vi "Lv_DEMO.vi"() -> ()   [LabVIEW 2019]
uses:
  C:/Users/Way/source/repos/MACOs.JY.ActorFramework/examples/Lv_DEMO/TestService.dll
  TestService.dll
  C:/Users/Way/source/repos/MACOs.JY.ActorFramework/examples/Lv_DEMO/MACOs.JY.ActorFramework.Implement.NetMQ.dll
  MACOs.JY.ActorFramework.Implement.NetMQ.dll
  C:/Users/Way/source/repos/MACOs.JY.ActorFramework/examples/net472_DEMO/bin/Debug/MACOs.JY.ActorFramework.Core.dll
  net472_DEMO/bin/Debug/MACOs.JY.ActorFramework.Core.dll
  C:/Users/Way/source/repos/MACOs.JY.ActorFramework/examples/net472_DEMO/bin/Debug/MACOs.JY.ActorFramework.Clients.dll
  net472_DEMO/bin/Debug/MACOs.JY.ActorFramework.Clients.dll
panel:
  out "error out":errorcluster
  in  "stop":bool
  in  "OK Button":bool
  out "Output String":string
  in  "Input String":string
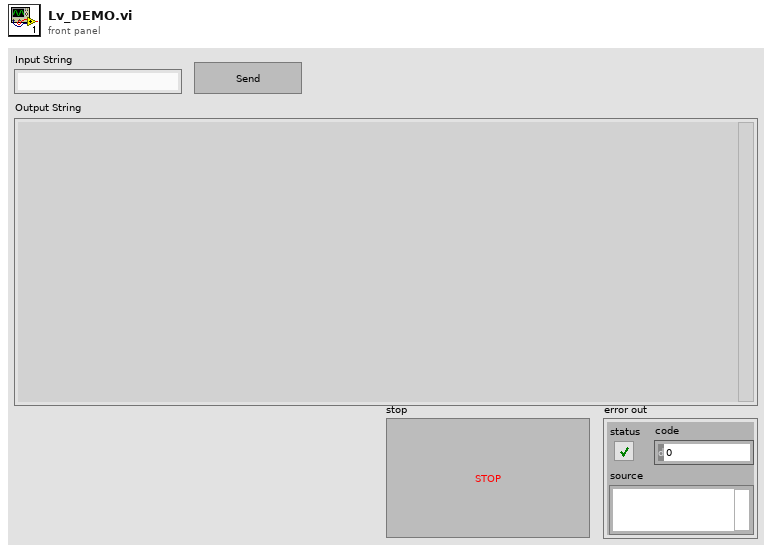
[diagram p1: front panel]
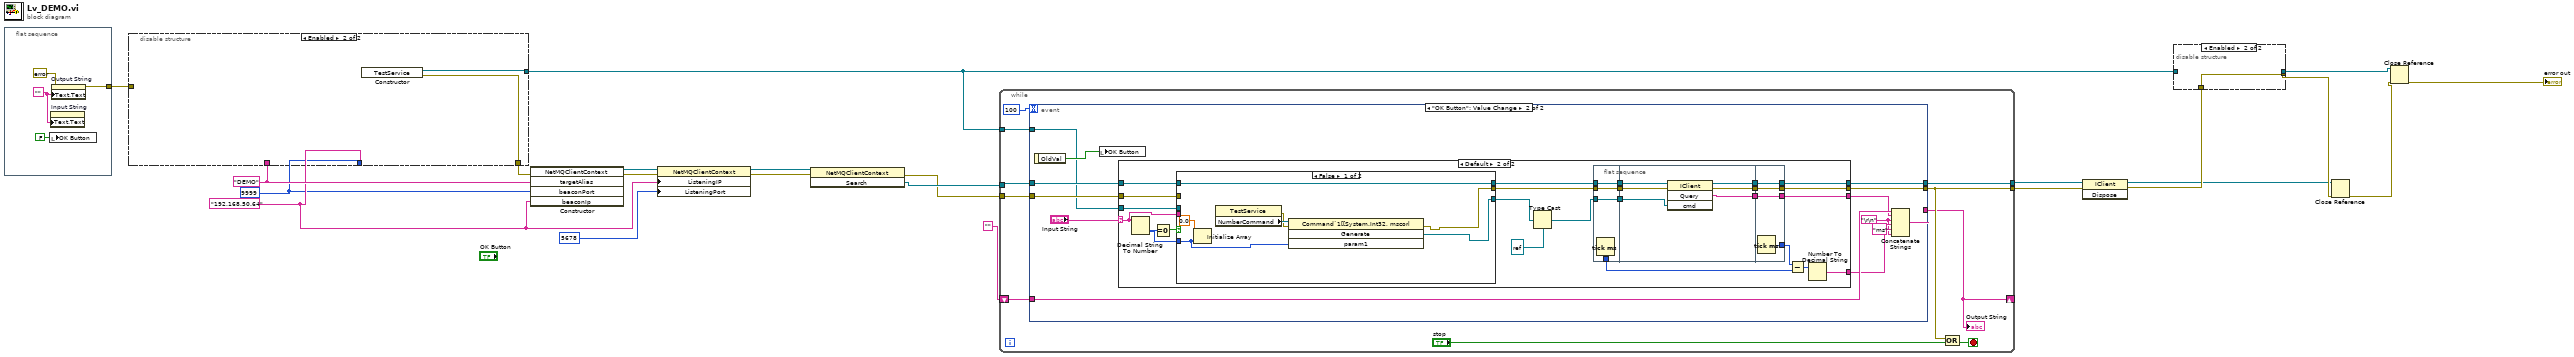
[diagram p0: block diagram]
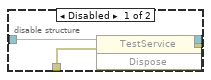
[diagram p2: hidden frame]
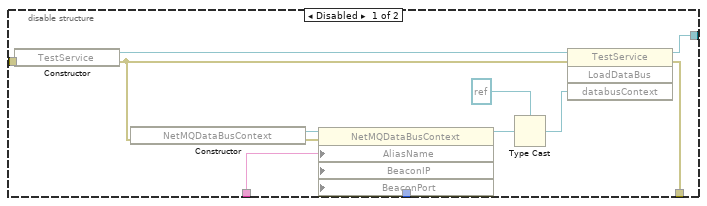
[diagram p3: hidden frame]
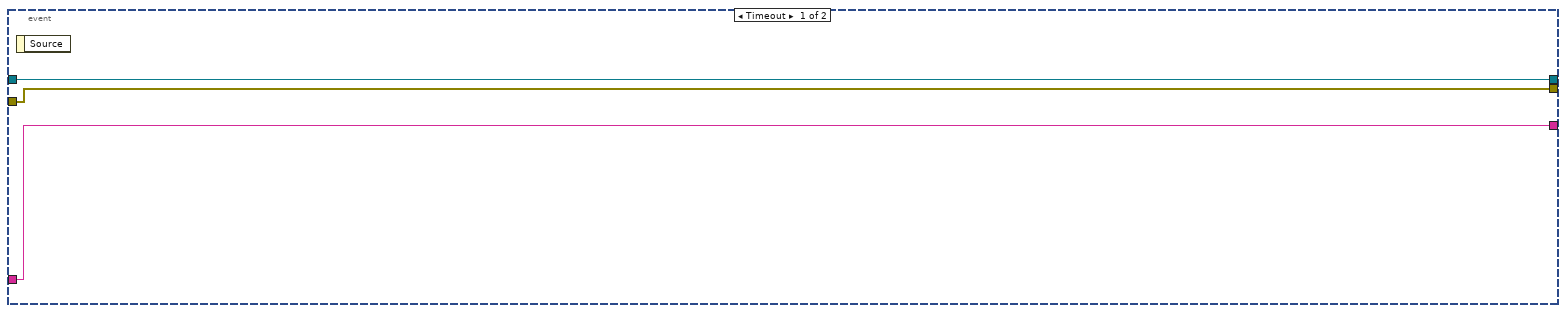
[diagram p4: hidden frame]
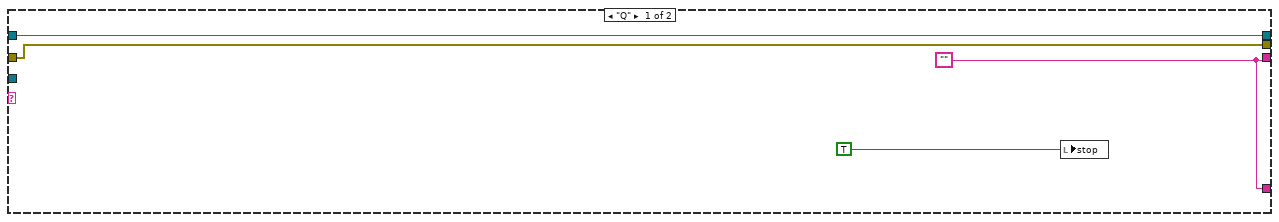
[diagram p5: hidden frame]
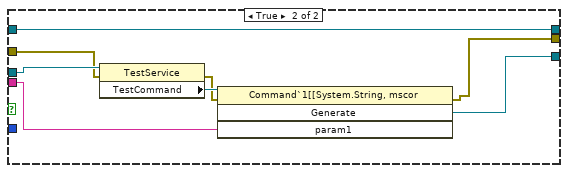
[diagram p6: hidden frame]
diagram:
  w2 = "192.168.50.64" ("alias")
  w11 = "DEMO" ("alias")
  w1 = 9999 ("port")
  n1 = flat-sequence {
    tunnel: [w26] -> w14
    frame #0 {
      w25 = ""
      n2 = local write "OK Button"(FALSE ("OK Button")) -> ()
      n3 = property on="Input String" class="Str"("Text.Text"=w25) -> ()  [unwired: 2 in, 2 out]
      n4 = property on="Output String" class="Str"(error in=errorcluster {"status"=FALSE, "code"=0, "source"=""} ("error in (no error)"), "Text.Text"=w25) -> (error out=w26:errorcluster)  [unwired: 1 in, 1 out]
    }
  }
  n5 = disable-structure shown="Enabled" {
    disable-tunnel: w14 -> [w39 _]
    disable-tunnel: [w37 w41] -> w12
    disable-tunnel: w11 -> [w30 _]
    disable-tunnel: [w29 w40] -> w10
    disable-tunnel: w2 -> [w28 _]
    disable-tunnel: w1 -> [w27 _]
    frame Disabled {
      n6 = constructor class="TestService"(error in=w39) -> (reference out=w38:refnum<k24>, error out=w36:errorcluster)  [unwired: 2 in, 1 out]
      n7 = constructor class="NetMQDataBusContext"(error in=w36) -> (reference out=w35:refnum<k24>, error out=w34:errorcluster)  [unwired: 2 in, 1 out]
      n8 = property class="NetMQDataBusContext"(reference=w35, error in=w34, "AliasName"=w30, "BeaconIP"=w28, "BeaconPort"=w27) -> (reference out=w33:refnum<k24>)  [unwired: 1 out]
      n9 = Type Cast(type=refnum<k24> refnum ("databusContext"), x=w33) -> (*(type *) &x=w32:refnum<k24>)
      n10 = invoke class="TestService" method="LoadDataBus"(reference=w38, error in=w36, "databusContext"=w32) -> (reference out=w37:refnum<k24>, error out=w29:errorcluster)  [unwired: 1 in, 2 out]
    }
    frame Enabled {
      n11 = constructor class="TestService"() -> (reference out=w41:refnum<k24>, error out=w40:errorcluster)  [unwired: 3 in, 1 out]
    }
  }
  n12 = constructor class="NetMQClientContext"(error in=w10, "targetAlias"=w11, "beaconPort"=w1, "beaconIp"=w2) -> (reference out=w7:refnum<k24>, error out=w6:errorcluster)  [unwired: 2 in, 4 out]
  n13 = property class="NetMQClientContext"(reference=w7, error in=w6, "ListeningIP"=w2, "ListeningPort"=5678) -> (reference out=w4:refnum<k24>, error out=w5:errorcluster)
  n14 = invoke class="NetMQClientContext" method="Search"(reference=w4, error in=w5) -> (error out=w8:errorcluster, "Search"=w9:refnum<k24>)  [unwired: 1 in, 1 out]
  n15 = while {
    tunnel: w9 -> [w50]
    tunnel: [w46] -> w22
    tunnel: [w49] -> w21
    tunnel: w8 -> [w45]
    shift-right: [w43] -> _
    shift-left: "" -> [w44]
    tunnel: w12 -> [w42]
    stop <- w47 stop-if-true
    n16 = event shown="[1] \"OK Button\": Value Change" {
      selector: _ -> [_ _]
      dyn-events: _ -> [_ _]
      timeout: 100 -> [_ _]
      tunnel: w50 -> [w54 w67]
      tunnel: [w52 w66] -> w46
      tunnel: [w54 w65] -> w49
      tunnel: w45 -> [w52 w64]
      tunnel: w44 -> [w53 w63]
      tunnel: [w53 w61] -> w43
      tunnel: w42 -> [_ w55]
      event Timeout {
        n17 = event-data() -> ()  [unwired: 1 in, 1 out]
      }
      event "OK Button": Value Change {
        w56 = "\r\n"
        n18 = event-data() -> ("OldVal"=w59:bool)  [unwired: 1 in]
        n19 = local write "OK Button"(w59) -> ()
        n20 = case shown="Default" "Input String" {
          selector: "Input String" -> [_ w87]
          tunnel: w67 -> [w69 w95]
          tunnel: [w71 w92] -> w66
          tunnel: [w69 w91] -> w65
          tunnel: w64 -> [w71 w90]
          tunnel: [w68 w89] -> w62
          tunnel: [w68 w79] -> w58
          tunnel: w55 -> [_ w75]
          frame "Q" {
            w68 = ""
            n21 = local write "stop"(TRUE ("stop")) -> ()
          }
          frame Default {
            n22 = Decimal String To Number(string=w87) -> (number=w86:i32)  [unwired: 2 in, 1 out]
            n23 = Equal To 0?(x=w86) -> (x = 0?=w88:bool)
            n24 = case shown="False" w88 {
              tunnel: w95 -> [w115 w124]
              tunnel: [w112 w118] -> w94
              tunnel: [w115 w124] -> w93
              tunnel: w90 -> [_ w122]
              tunnel: w87 -> [_ w120]
              tunnel: w86 -> [w110 _]
              tunnel: [w111 w117] -> w74
              tunnel: w75 -> [_ w123]
              frame False {
                n25 = Initialize Array(0.0, w110) -> ()  [unwired: 1 out]
                n26 = property class="TestService"() -> (error out=w113:errorcluster, "NumberCommand"=w114:refnum<k24>)  [unwired: 2 in, 1 out]
                n27 = invoke class="Command`1[[System.Int32, mscorl" method="Generate"(reference=w114, error in=w113, "param1"=w110) -> (error out=w112:errorcluster, "Generate"=w111:refnum<k24>)  [unwired: 1 in, 2 out]
              }
              frame True {
                n28 = property class="TestService"(reference=w123, error in=w122) -> (error out=w119:errorcluster, "TestCommand"=w121:refnum<k24>)  [unwired: 1 out]
                n29 = invoke class="Command`1[[System.String, mscor" method="Generate"(reference=w121, error in=w119, "param1"=w120) -> (error out=w118:errorcluster, "Generate"=w117:refnum<k24>)  [unwired: 1 in, 2 out]
              }
            }
            n30 = Type Cast(type=refnum<k24> refnum ("cmd"), x=w74) -> (*(type *) &x=w73:refnum<k24>)
            n31 = flat-sequence {
              tunnel: w93 -> [w98]
              tunnel: w94 -> [w99]
              tunnel: [w99] -> w84
              tunnel: [w98] -> w83
              tunnel: [w97] -> w81
              tunnel: [w96] -> w78
              tunnel: w73 -> [w96]
              tunnel: [w103] -> w85
              tunnel: w84 -> [w101]
              tunnel: w83 -> [w105]
              tunnel: w78 -> [w100]
              tunnel: [w104] -> w77
              tunnel: [w102] -> w76
              tunnel: [w107] -> w89
              tunnel: [w108] -> w91
              tunnel: [w109] -> w92
              tunnel: w85 -> [w109]
              tunnel: [w106] -> w82
              tunnel: w77 -> [w107]
              tunnel: w76 -> [w108]
              frame #0 {
                n32 = Tick Count (ms)() -> (millisecond timer value=w97:u32)
              }
              frame #1 {
                n33 = invoke class="IClient" method="Query"(reference=w105, error in=w101, "cmd"=w100) -> (reference out=w102:refnum<k24>, error out=w103:errorcluster, "Query"=w104:string)  [unwired: 1 in, 1 out]
              }
              frame #2 {
                n34 = Tick Count (ms)() -> (millisecond timer value=w106:u32)
              }
            }
            n35 = Subtract(x=w82, y=w81) -> (x-y=w80:u32)
            n36 = Number To Decimal String(number=w80) -> (decimal integer string=w79:string)  [unwired: 1 in]
          }
        }
        n37 = Concatenate Strings(w63, w62, w56, w58, "ms" ("string"), w56) -> (w61:string)
      }
    }
    "Output String" <- w43
    n38 = Compound Arithmetic op=OR(w46, "stop") -> (w47:bool)
  }
  n39 = invoke class="IClient" method="Dispose"(reference=w21, error in=w22) -> (reference out=w15:refnum<k24>, error out=w19:errorcluster)  [unwired: 1 in, 1 out]
  n40 = disable-structure shown="Enabled" {
    disable-tunnel: w19 -> [w128 w129]
    disable-tunnel: [w127 w129] -> w18
    disable-tunnel: [w126 _] -> w16
    disable-tunnel: w12 -> [w125 _]
    frame Disabled {
      n41 = invoke class="TestService" method="Dispose"(reference=w125, error in=w128) -> (reference out=w126:refnum<k24>, error out=w127:errorcluster)  [unwired: 1 in, 1 out]
    }
    frame Enabled {
    }
  }
  n42 = Close Reference(reference=w15, error in (no error)=w18) -> (error out=w20:errorcluster)
  n43 = Close Reference(reference=w16, error in (no error)=w20) -> (error out=→"error out":errorcluster)
